vi "SvgDoc Raster Draw Bitmap.vi"(8 "error in (no error)":errorcluster, 9 "rasterHeight":i32, 10 "rasterWidth":i32, 11 ".NET Refnum in":refnum<k24>) -> (0 "error out":errorcluster, 2 "Bitmap":refnum<k24>, 3 "reference out":refnum<k24>)   [LabVIEW 2020, in "SvgDotNet.lvlib"]
uses:
  SvgDotNet.lvlib
  C:/Users/huipeng8/Desktop/SVG.NET/Svg.dll
  Svg.dll
  System.Drawing
panel:
  # "Connector Pane"
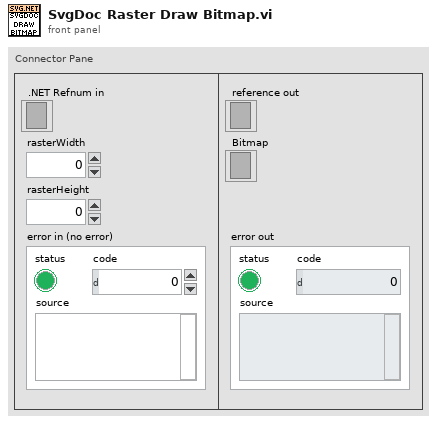
[diagram p1: front panel]
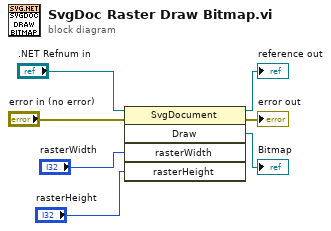
[diagram p0: block diagram]
diagram:
  n1 = invoke class="SvgDocument" method="Draw"(reference=".NET Refnum in", error in="error in (no error)", "rasterWidth"="rasterWidth", "rasterHeight"="rasterHeight") -> (reference out=→"reference out":refnum<k24>, error out=→"error out":errorcluster, "Draw"=→"Bitmap":refnum<k24>)  [unwired: 1 in, 2 out]
